vi "Scale_EU_to_RaW.vi"(10 "ConfigScale":T1={"scale [EU/RAW]"=1.0, "offset [EU]"=0.0} {"offset [EU]" format="%0.2f"; "scale [EU/RAW]" format="%0.2f"}, 11 "EU":dbl) -> (3 "RAW":dbl)   [LabVIEW 2019]
uses:
  TypeDef/Config_Scale.ctl
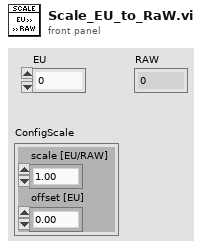
[diagram p1: front panel]
types:
  T1 = typedef "Config_Scale.ctl" = cluster{"scale [EU/RAW]":dbl, "offset [EU]":dbl}
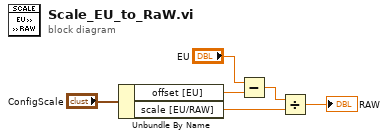
[diagram p0: block diagram]
diagram:
  n1 = Unbundle By Name("ConfigScale") -> ("offset [EU]"=w1:dbl, "scale [EU/RAW]"=w3:dbl)
  n2 = Subtract(x="EU", y=w1) -> (x-y=w4:dbl)
  n3 = Divide(x=w4, y=w3) -> (x/y=→"RAW":dbl)
